vi "defineCircleParameters.vi"(0 "Game in":refnum<class "Game.lvclass">, 1 "Dest_array in":T1(array[cluster]), 3 "robotModel":dbl[][](array[numeric]), 4 "v_ang_curve":dbl format="%#_13g", 5 "error in (no error)":errorcluster, 6 "angle":dbl, 7 "L":dbl format="%#_13g", 8 "distRobotNextDest":dbl format="%0.2f", 9 "est_vel":dbl[](array[numeric]), 11 "max_v_sent":dbl=0.2 format="%#_13g", 13 "delta":dbl=0.2 format="%#_13g") -> (14 "Game out":refnum<class "Game.lvclass">, 15 "L out":dbl, 18 "velToBeginCircle":dbl, 19 "error out":errorcluster)   [LabVIEW 2021, in "Game.lvclass"]
uses:
  Game.lvclass
panel:
  out "degree":dbl
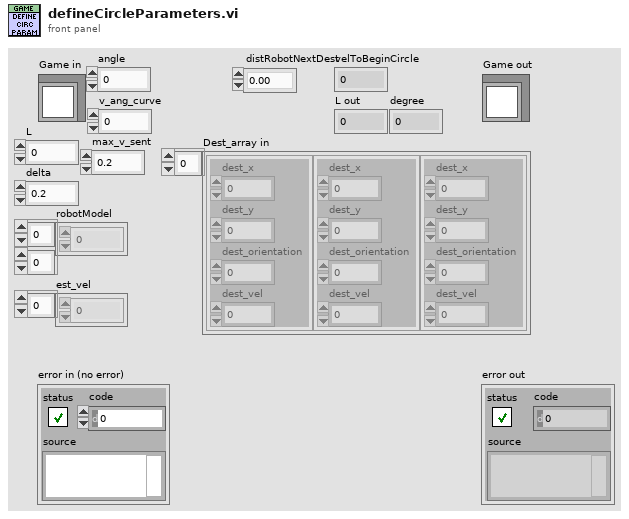
[diagram p1: front panel]
types:
  T1 = cluster{"dest_x":dbl, "dest_y":dbl, "dest_orientation":dbl, "dest_vel":dbl}[]
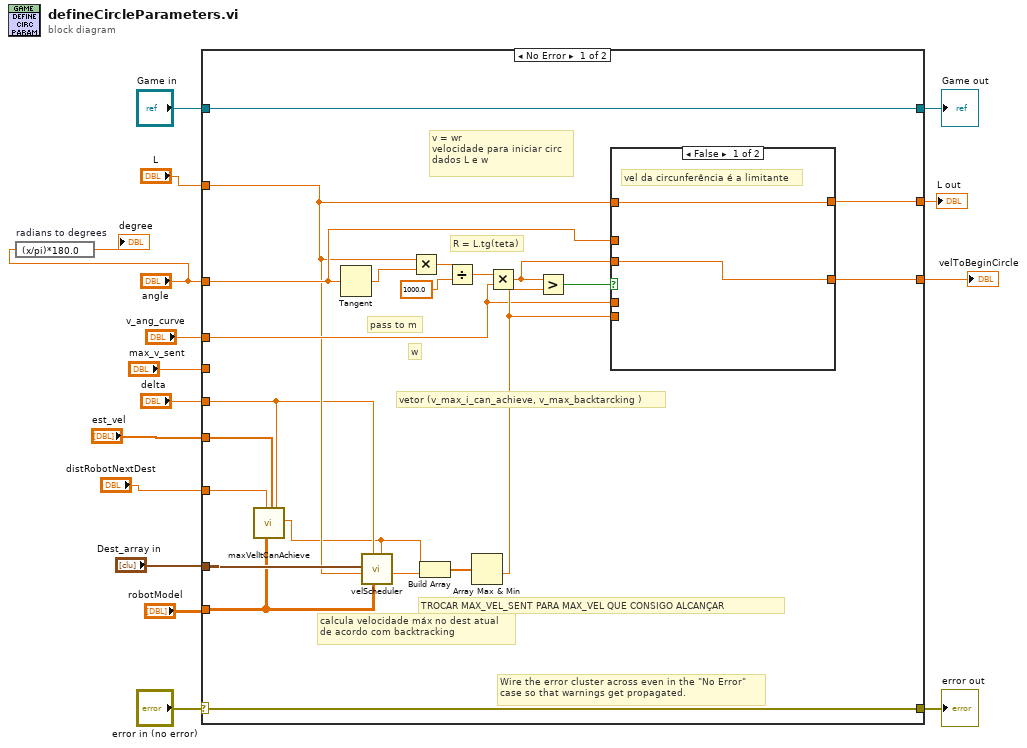
[diagram p0: block diagram]
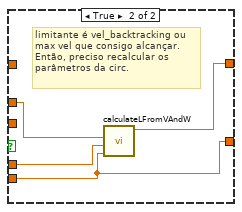
[diagram p2: hidden frame]
diagram:
  n1 = expression code="(x/pi)*180.0" "radians to degrees"("angle") -> (→"degree":dbl)
  n2 = case shown="No Error" "error in (no error)" {
    selector: "error in (no error)" -> [w37 w46]
    tunnel: [w37 w46] -> w15
    tunnel: [w38 w45] -> w13
    tunnel: "Game in" -> [w38 w45]
    tunnel: "angle" -> [w30 _]
    tunnel: "v_ang_curve" -> [w29 _]
    tunnel: [w33 _] -> w11
    tunnel: "L" -> [w22 _]
    tunnel: [w32 _] -> w9
    tunnel: "Dest_array in" -> [w25 _]
    tunnel: "max_v_sent" -> [_ _]
    tunnel: "delta" -> [w21 _]
    tunnel: "robotModel" -> [w18 _]
    tunnel: "est_vel" -> [w20 _]
    tunnel: "distRobotNextDest" -> [w19 _]
    frame No Error {
      # "calcula velocidade máx no dest atual\nde acordo com backtracking"
      # "TROCAR MAX_VEL_SENT PARA MAX_VEL QUE CONSIGO ALCANÇAR"
      # "vetor (v_max_i_can_achieve, v_max_backtarcking )"
      # "pass to m"
      # "v = wr\nvelocidade para iniciar circ\ndados L e w"
      # "w"
      # "R = L.tg(teta)"
      # "Wire the error cluster across even in the \"No Error\"\ncase so that warnings get propagated."
      n3 = call "maxVelItCanAchieve.vi"("distRobotNextDest"=w19, "robotModel"=w18, "est_vel"=w20, "delta"=w21) -> ("maxVelPossibleAtNextDest"=w17:dbl)  [unwired: 13 in, 2 out]
      n4 = Tangent(1:w30) -> (0:w36:dbl)
      n5 = call "velScheduler.vi"("max_v_sent"=w17, "robotModel"=w18, "delta"=w21, "L"=w22, "Dest_array in"=w25) -> ("backtracking_max_dest_vel_to_next_dest"=w24:dbl)  [unwired: 3 in, 3 out]
      n6 = Multiply(x=w22, y=w36) -> (x*y=w28:dbl)
      n7 = Build Array(w17, w24) -> (w23:dbl[])
      n8 = Divide(x=w28, y=1000.0) -> (x/y=w27:dbl)
      n9 = Array Max & Min(array=w23) -> (min value=w31:dbl)  [unwired: 3 out]
      n10 = Multiply(x=w27, y=w29) -> (x*y=w34:dbl)
      n11 = Greater?(x=w34, y=w31) -> (0:w35:bool)
      n12 = case shown="False" w35 {
        tunnel: w34 -> [w40 _]
        tunnel: [w40 w41] -> w33
        tunnel: w22 -> [w39 _]
        tunnel: [w39 w44] -> w32
        tunnel: w31 -> [_ w41]
        tunnel: w30 -> [_ w43]
        tunnel: w29 -> [_ w42]
        frame False {
          # "vel da circunferência é a limitante"
        }
        frame True {
          # "limitante é vel_backtracking ou\nmax vel que consigo alcançar.\nEntão, preciso recalcular os \nparâmetros da circ."
          n13 = call "calculateLFromVAndW.vi"("v_tang_curve"=w41, "v_ang_curve"=w42, "angle"=w43) -> ("L"=w44:dbl)  [unwired: 8 in]
        }
      }
    }
    frame Error {
    }
  }
  "error out" <- w15
  "Game out" <- w13
  "velToBeginCircle" <- w11
  "L out" <- w9
